vi "Set Front Panel Inhibit Mode (RS-232).vi"(8 "error in (no error)":errorcluster, 10 "Front Panel Inhibit Mode (Local)":T1, 11 "VISA resource name":refnum<visa-resource-name>) -> (0 "error out":errorcluster, 3 "VISA resource name out":refnum<visa-resource-name>)   [LabVIEW 2013, in "SRS SR400.lvlib"]
doc: "<B>MI j</B>\n\nThe MI command sets the front panel inhibit mode. j is a required parameter from 0 to 2.\n\n<B>j</B> <B>Mode</B>\n0 Local: all front panel controls are operative\n1 Remote: front panel controls are not operative. The LOCAL (COM) key returns the status to local.\n2 Lock-out: front panel controls are not operative. No key returns the status to local. Another MI command is needed to return to local.\n\nThe MI command may only be sent via the RS-232 interface. The GPIB interface uses REN, LLO, and GTL to set the front panel mode."
uses:
  <instrlib>/SRS SR400/SRS SR400.lvlib
  <instrlib>/SRS SR400/Public/Typedefs/Front Panel Inhibit Mode.ctl
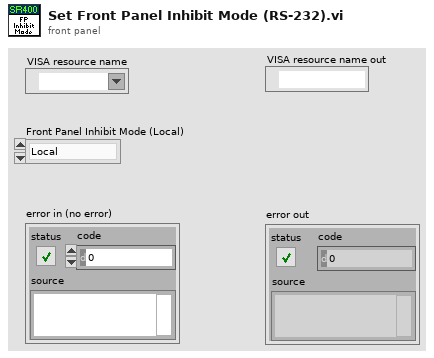
[diagram p1: front panel]
types:
  T1 = typedef "SRS SR400.lvlib/Front Panel Inhibit Mode.ctl" = enum16{"Local", "Remote", "Lock-out"}
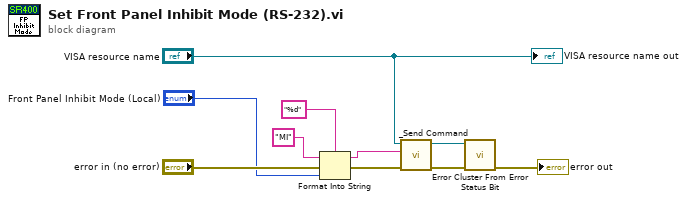
[diagram p0: block diagram]
diagram:
  n1 = Format Into String(format string="%d", initial string="MI", error in="error in (no error)", "Front Panel Inhibit Mode (Local)") -> (resulting string=w5:string, error out=w6:errorcluster)
  n2 = call <instrlib>:"_Send Command.vi"("error in (no error)"=w6, "Command"=w5, "VISA resource name"="VISA resource name") -> ("error out"=w3:errorcluster, "VISA resource name out"=w1:refnum<visa-resource-name>)  [unwired: 6 in, 1 out]
  n3 = call <instrlib>:"Error Cluster From Error Status Bit.vi"("error in (no error)"=w3, "VISA resource name"=w1) -> ("error out"=→"error out":errorcluster)  [unwired: 8 in, 1 out]
  "VISA resource name out" <- "VISA resource name"
